vi "read_NP_Dop_flow.vi"() -> (0 "N/P Dopant DA Switch":bool, 1 "N/P_Dop Flow 3":dbl, 2 "N/P_Dop Flow 2 or 4":dbl, 3 "N/P_Dop Flow 1":dbl)   [LabVIEW 2011]
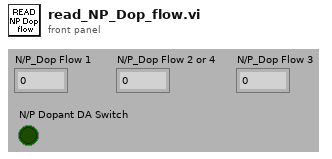
[diagram p1: front panel]
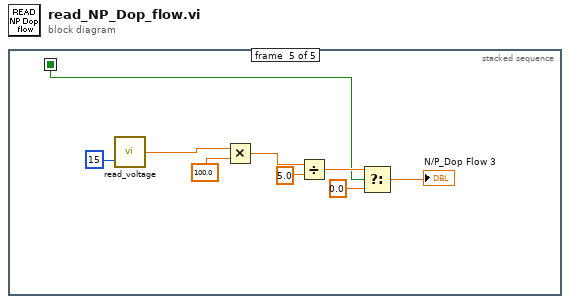
[diagram p0: block diagram]
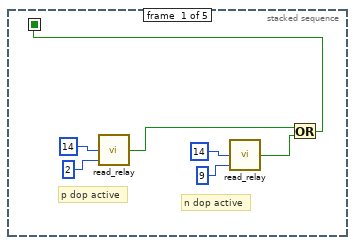
[diagram p2: hidden frame]
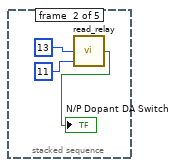
[diagram p3: hidden frame]
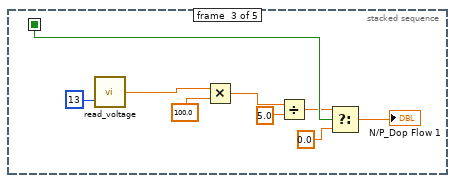
[diagram p4: hidden frame]
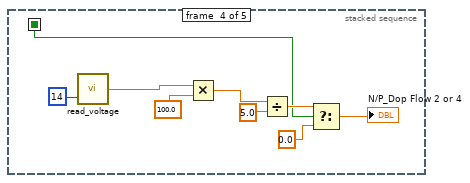
[diagram p5: hidden frame]
diagram:
  n1 = stacked-sequence {
    seq-local: [w1 _ _ _ _] -> [_ _ w14 w22 w30]
    frame #0 {
      # "n dop active"
      # "p dop active"
      n2 = call "read_relay.vi"("Relay"=2, "Slot"=14) -> ("Relay Status"=w3:bool)  [unwired: 1 out]
      n3 = call "read_relay.vi"("Relay"=9, "Slot"=14) -> ("Relay Status"=w2:bool)  [unwired: 1 out]
      n4 = Or(x=w3, y=w2) -> (x .or. y?=w1:bool)
    }
    frame #1 {
      n5 = call "read_relay.vi"("Relay"=11, "Slot"=13) -> ("Relay Status"=→"N/P Dopant DA Switch":bool)  [unwired: 1 out]
    }
    frame #2 {
      n6 = call "read_voltage.vi"("Channel"=13) -> ("Voltage"=w15:dbl)  [unwired: 1 in]
      n7 = Multiply(x=w15, y=100.0) -> (x*y=w17:dbl)
      n8 = Divide(x=w17, y=5.0) -> (x/y=w13:dbl)
      n9 = Select(t=w13, s=w14, f=0.0) -> (s? t:f=→"N/P_Dop Flow 1":dbl)
    }
    frame #3 {
      n10 = call "read_voltage.vi"("Channel"=14) -> ("Voltage"=w28:dbl)  [unwired: 1 in]
      n11 = Multiply(x=w28, y=100.0) -> (x*y=w26:dbl)
      n12 = Divide(x=w26, y=5.0) -> (x/y=w23:dbl)
      n13 = Select(t=w23, s=w22, f=0.0) -> (s? t:f=→"N/P_Dop Flow 2 or 4":dbl)
    }
    frame #4 {
      n14 = call "read_voltage.vi"("Channel"=15) -> ("Voltage"=w33:dbl)  [unwired: 1 in]
      n15 = Multiply(x=w33, y=100.0) -> (x*y=w35:dbl)
      n16 = Divide(x=w35, y=5.0) -> (x/y=w32:dbl)
      n17 = Select(t=w32, s=w30, f=0.0) -> (s? t:f=→"N/P_Dop Flow 3":dbl)
    }
  }
